vi "Core.vi"(8 "error in (no error)":errorcluster, 10 "Actor in":refnum<class "Actor.lvclass">, 11 "List Instruments Msg in":refnum<class "List Driver Aliases Msg.lvclass">) -> (0 "error out":errorcluster, 1 "Data":refnum<class "Data.lvclass">, 2 "Actor out":refnum<class "Actor.lvclass">, 3 "List Instruments Msg out":refnum<class "List Driver Aliases Msg.lvclass">)   [LabVIEW 2020, in "Instrument Handler.lvlib" / "List Driver Aliases Msg.lvclass"]
doc: "Core of the Reponse Msg. Put the active code here.\n\nThis implementation does nothing."
uses:
  List Driver Aliases Msg.lvclass
  PPL/HDH.Data.Generic.lvlibp/Data.lvclass
  PPL/HDH.Actor Framework.Core.Actor.lvlibp/1abvi3w/vi.lib/ActorFramework/Actor/Actor.lvclass
  Instrument Handler/Instrument Handler.lvclass
  C:/Current projects/WS/PPL/HDH.Actor Framework.Core.Actor.lvlibp/1abvi3w/vi.lib/ActorFramework/Actor/Actor.lvclass
  Data/Instrument Alias Data/Instrument Alias Data.lvclass/Instrument Alias Data.ctl
  Data/Instrument Alias Data/Instrument Alias Data.lvclass
  C:/Current projects/WS/PPL/HDH.Data.Generic.lvlibp/Data.lvclass
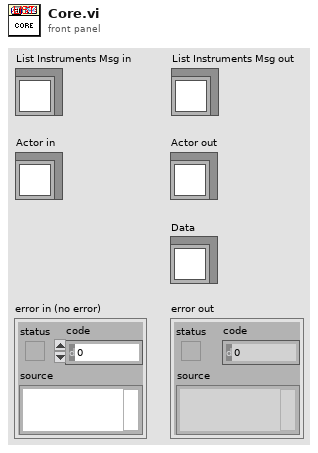
[diagram p1: front panel]
types:
  T1 = typedef "Instrument Handler.lvlib/Ctl_DriverAliasElement.ctl" = cluster{"Driver Name":string, "Alias Array":string[]}
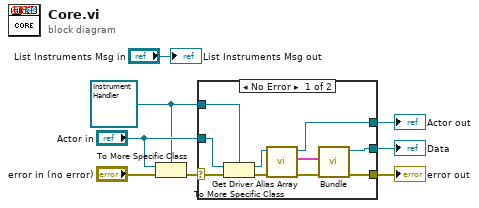
[diagram p0: block diagram]
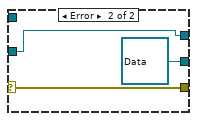
[diagram p2: hidden frame]
diagram:
  w4 = refnum<class "Instrument Handler.lvclass"> refnum ("Instrument Handler.lvlib:Instrument Handler.lvclass")
  n1 = To More Specific Class(target class=w4, reference="Actor in", error in="error in (no error)") -> (error out=w7:errorcluster)  [unwired: 1 out]
  n2 = case shown="No Error" w7 {
    selector: w7 -> [w18 w21]
    tunnel: [w11 w21] -> w6
    tunnel: [w13 w20] -> w2
    tunnel: "Actor in" -> [w17 w20]
    tunnel: w4 -> [w16 _]
    tunnel: [w10 refnum<class "Data.lvclass"> refnum ("Data")] -> w1
    frame No Error {
      n3 = To More Specific Class(target class=w16, reference=w17, error in=w18) -> (specific class reference=w15:refnum<class "Instrument Handler.lvclass">, error out=w14:errorcluster)
      n4 = call "Get Driver Alias Array.vi"("error in (no error)"=w14, "Instrument Handler in"=w15) -> ("error out"=w12:errorcluster, "Driver Alias Array"=w9:T1[], "Instrument Handler out"=w13:refnum<class "Instrument Handler.lvclass">)  [unwired: 7 in]
      n5 = call "Bundle.vi"("error in"=w12, "Instrument Alias Array"=w9) -> ("error out"=w11:errorcluster, "Instrument Alias Data out"=w10:refnum<class "Instrument Alias Data.lvclass">)  [unwired: 8 in]
    }
    frame Error {
    }
  }
  "error out" <- w6
  "Actor out" <- w2
  "Data" <- w1
  "List Instruments Msg out" <- "List Instruments Msg in"
